vi "EN1 VIs.vi"   [LabVIEW 2019]
uses:
  <vilib>/httpClient/LabVIEWHTTPClient.lvlib
  <vilib>/httpClient/POSTBuffer.vi
  <vilib>/httpClient/PUTBuffer.vi
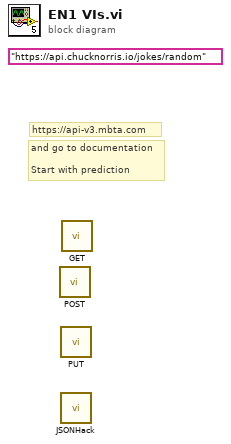
[diagram p0: block diagram]
diagram:
  (unwired) "https://api.chucknorris.io/jokes/random"
  # "and go to documentation\n\nStart with prediction"
  # "https://api-v3.mbta.com"
  n1 = call-poly <vilib>:"POST.vi"() -> ()  [unwired: 12 in, 4 out]
  n2 = call-poly <vilib>:"PUT.vi"() -> ()  [unwired: 12 in, 4 out]
  n3 = call "JSONHack.vi"() -> ()  [unwired: 8 in, 4 out]
  n4 = call <vilib>:"GET.vi"() -> ()  [unwired: 12 in, 4 out]
